vi "Time Proportioning [array] v3.vi"(1 "Now (mS)":u32, 2 "Cycle Time (mS)":dbl=5000.0, 3 "On Time (%)":dbl[](array[numeric]) format="%.2f") -> (0 "Relay Output":bool[](array[boolean]))   [LabVIEW 2020]
doc: "This vi will individually time proportion the bits of a boolean array. That is it will turn each bit on for the requested percentage (OnTime (%)) of each duty cycle (Cycle Time (Sec)). It is designed to run within the While loop of a larger control application. The longer the cycle time, and the shorter the loop delay, the better for timing accuracy. Cycle times less than 5 seconds will probably lead to unacceptable jitter in On Time accuracy due to Windows timing latency.\nW.J. Gilbert 8/4/2000, wgilbert@minn.net"
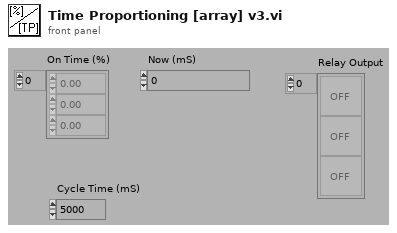
[diagram p1: front panel]
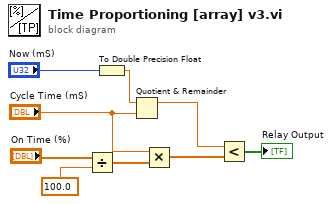
[diagram p0: block diagram]
diagram:
  n1 = Divide(x="On Time (%)", y=100.0) -> (x/y=w7:dbl[])
  n2 = To Double Precision Float(number="Now (mS)") -> (double precision float=w1:dbl)
  n3 = Quotient & Remainder(x=w1, y="Cycle Time (mS)") -> (x-y*floor(x/y)=w4:dbl)  [unwired: 1 out]
  n4 = Multiply(x="Cycle Time (mS)", y=w7) -> (x*y=w6:dbl[])
  n5 = Less?(x=w4, y=w6) -> (x < y?=→"Relay Output":bool[])
